vi "sub_Extract_Packet_Boundaries - G.vi"(5 "Thresholded Signal":bool[](array[boolean])) -> (0 "packet_start_loc":i32[](array[numeric]), 3 "packet_end_loc":i32[](array[numeric]), 4 "Packet Detection Error?":bool)   [LabVIEW 2023]
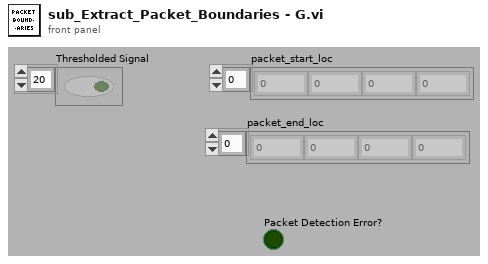
[diagram p1: front panel]
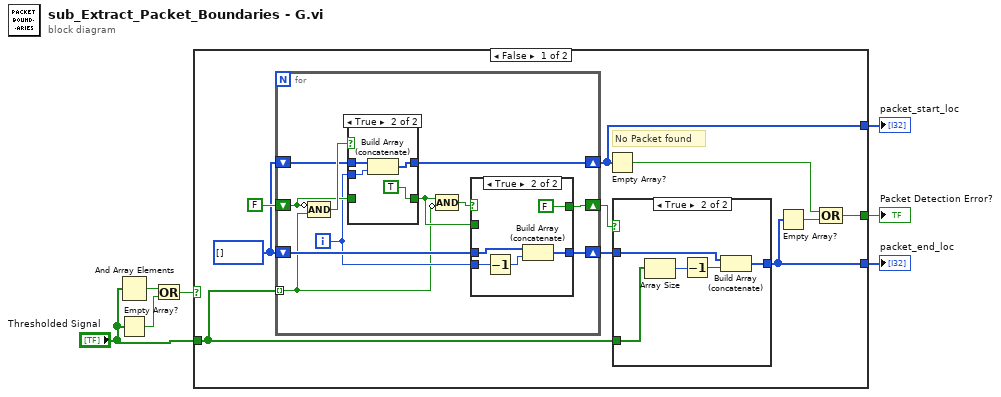
[diagram p0: block diagram]
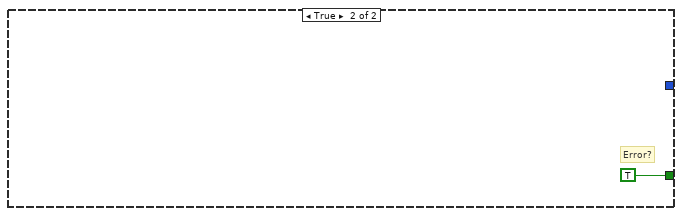
[diagram p5: hidden frame]
diagram:
  n1 = And Array Elements(Boolean array="Thresholded Signal") -> (logical AND=w2:bool)
  n2 = Empty Array?(array="Thresholded Signal") -> (empty?=w4:bool)
  n3 = Or(x=w2, y=w4) -> (x .or. y?=w3:bool)
  n4 = case shown="False" w3 {
    tunnel: "Thresholded Signal" -> [w8 _]
    tunnel: [w16 TRUE] -> w5
    tunnel: [w9 _] -> w6
    tunnel: [w10 _] -> w7
    frame False {
      w13 = i32[] []
      # "No Packet found"
      n5 = for {
        shift-right: [w26] -> w12
        shift-left: FALSE -> [w28]
        shift-right: [w32] -> w9
        shift-left: w13 -> [w33]
        shift-right: [w29] -> w11
        shift-left: w13 -> [w30]
        tunnel: w8 -> [w24] mode=indexing
        i -> [w25]
        n6 = Compound Arithmetic op=AND(invert w28, w24) -> (w34:bool)
        n7 = case shown="True" w34 {
          tunnel: w33 -> [w43 w47]
          tunnel: [w43 w46] -> w32
          tunnel: [w42 TRUE] -> w27
          tunnel: w25 -> [_ w44]
          tunnel: w28 -> [w42 _]
          frame False {
          }
          frame True {
            n8 = Build Array (concatenate)(w47, w44) -> (w46:i32[])
          }
        }
        n9 = Compound Arithmetic op=AND(w27, invert w24) -> (w31:bool)
        n10 = case shown="True" w31 {
          tunnel: w30 -> [w36 w41]
          tunnel: [w36 w40] -> w29
          tunnel: [w35 FALSE] -> w26
          tunnel: w25 -> [_ w38]
          tunnel: w27 -> [w35 _]
          frame False {
          }
          frame True {
            n11 = Decrement(x=w38) -> (x-1=w37:i32)
            n12 = Build Array (concatenate)(w41, w37) -> (w40:i32[])
          }
        }
      }
      n13 = Empty Array?(array=w9) -> (empty?=w17:bool)
      n14 = case shown="True" w12 {
        tunnel: w11 -> [w18 w23]
        tunnel: [w18 w21] -> w10
        tunnel: w8 -> [_ w19]
        frame False {
        }
        frame True {
          n15 = Array Size(array=w19) -> (size(s)=w20:i32)
          n16 = Decrement(x=w20) -> (x-1=w22:i32)
          n17 = Build Array (concatenate)(w23, w22) -> (w21:i32[])
        }
      }
      n18 = Empty Array?(array=w10) -> (empty?=w15:bool)
      n19 = Compound Arithmetic op=OR(w17, w15) -> (w16:bool)
    }
    frame True {
      # "Error?"
    }
  }
  "Packet Detection Error?" <- w5
  "packet_end_loc" <- w7
  "packet_start_loc" <- w6
